vi "Kill Process.vi"(4 "error in (no error)":errorcluster, 7 "Name of Process to kill (\"\")":string) -> (0 "error out":errorcluster)   [LabVIEW 2011]
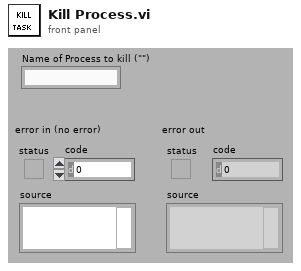
[diagram p1: front panel]
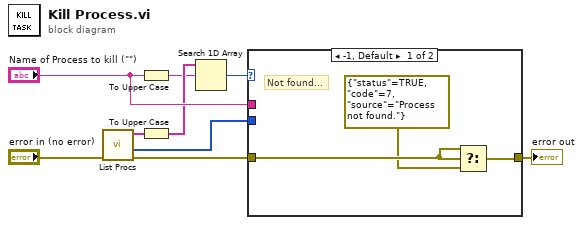
[diagram p0: block diagram]
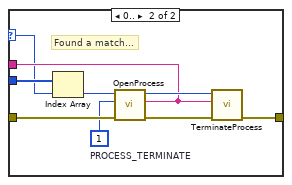
[diagram p2: hidden frame]
diagram:
  n1 = call "List Procs.vi"("error in (no error)"="error in (no error)") -> ("error out"=w4:errorcluster, "ProcId's"=w6:i32[], "ProcessNames"=w5:string[])  [unwired: 4 out]
  n2 = To Upper Case(1:"Name of Process to kill (\"\")") -> (0:w2:string)
  n3 = To Upper Case(1:w5) -> (0:w3:string[])
  n4 = Search 1D Array(1D array=w3, element=w2) -> (index of element=w1:i32)  [unwired: 1 out]
  n5 = case shown="-1, Default" w1 {
    selector: w1 -> [_ w13]
    tunnel: w6 -> [_ w19]
    tunnel: [w11 w17] -> w8
    tunnel: w4 -> [w12 w16]
    tunnel: "Name of Process to kill (\"\")" -> [_ w14]
    frame -1, Default {
      # "Not found..."
      n6 = Select(t=w12, s=w12, f=errorcluster {"status"=TRUE, "code"=7, "source"="Process not found."} ("error out")) -> (s? t:f=w11:errorcluster)
    }
    frame 0.. {
      w15 = 1  # PROCESS_TERMINATE
      # "Found a match..."
      n7 = Index Array(array=w19, index=w13) -> (element=w18:i32)
      n8 = call "OpenProcess.vi"("process name"=w14, "error in (no error)"=w16, "dwDesiredAccesses (0)"=w15, "dwProcessId (0)"=w18) -> ("error out"=w20:errorcluster, "hProcess"=w21:i32)  [unwired: 1 in, 1 out]
      n9 = call "TerminateProcess.vi"("error in (no error)"=w20, "process name"=w14, "hProcess"=w21) -> ("error out"=w17:errorcluster)  [unwired: 4 out]
    }
  }
  "error out" <- w8
